vi "AlliGator Phasor Color Map Picker.vi"() -> ()   [LabVIEW 2021, in "AlliGator Phasor Plot Color Map.lvlib"]
doc: "UI to define the vertices of a color map (using cursors) as well as their colors."
uses:
  AlliGator Phasor Plot Color Map.lvlib
  AlliGator Phasor Color Map User Event List.ctl
  5d2066e6-2ae8-4eda-ab8b-78fd27cf9e73.vi
  Phasor/Phasor.lvlib
  Graphs/XY Graph/XY Graph Add-Ons.lvlib
  Error/Error.lvlib
  Arrays/Arrays.lvlib
panel:
  in  "Background":u32(colorbox)=16448250
  in  "Plot Color":u32(colorbox)
  in  "Show Cursor Axes":bool=TRUE
  in  "Decay Range Exponent":dbl=1.0
  in  "Color Array":u32[](array[colorbox])
  out "Color Map Picker Graph":cluster{"X Array":dbl[], "Y Array":dbl[]}[](graph)=[{"X Array"=[1.0, 0.9997482711915926, 0.9989933382359422, 0.9977359612865423, 0.9959774064153977, 0.9937194443381971, 0.9909643486313533, 0.9877148934427036, 0.9839743506981782, 0.9797464868072487, 0.9750355588704727, 0.9698463103929542, 0.9641839665080363, 0.9580542287160347, 0.9514632691433107, 0.9444177243274617, 0.9369246885348925, 0.9289917066174885, 0.9206267664155906, 0.9118382907149164, 0.9026351287655293, 0.8930265473713938, 0.883022221559489, 0.8726322248378774, 0.861867019052535, 0.8507374438531606, 0.8392547057785661, 0.8274303669726426, 0.8152763335422613, 0.8028048435688333, 0.7900284547855991, 0.7769600319330552, 0.7636127338052512, 0.75, 0.7361355373863413, 0.722033306302887, 0.707707506500943, 0.6931725628465641, 0.6784431107959357, 0.6635339816587105, 0.648460187664137, 0.633236906845017, 0.6178794677547131, 0.6024033340325947, 0.5868240888334646, 0.5711574191366419, 0.5554190999505048, 0.5396249784283934, 0.5237909579118704, 0.5079329819174031, 0.4920670180825951, 0.47620904208812787, 0.4603750215716047, 0.4445809000494934, 0.4288425808633563, 0.4131759111665336, 0.39759666596740345, 0.38212053224528514, 0.3667630931549812, 0.35153981233586123, 0.3364660183412878, 0.32155688920406267, 0.30682743715343425, 0.2922924934990553, 0.2779666936971116, 0.2638644626136573, 0.24999999999999878, 0.2363872661947476, 0.22303996806694376, 0.20997154521439987, 0.1971951564311657, 0.18472366645773786, 0.17256963302735667, 0.16074529422143313, 0.1492625561468387, 0.1381329809474643, 0.12736777516212205, 0.1169777784405105, 0.1069734526286058, 0.0973648712344703, 0.08816170928508327, 0.07937323358440912, 0.07100829338251125, 0.06307531146510731, 0.055582275672538095, 0.04853673085668925, 0.041945771283965094, 0.035816033491963606, 0.030153689607045786, 0.02496444112952728, 0.020253513192751316, 0.016025649301821876, 0.012285106557296477, 0.009035651368646702, 0.006280555661802856, 0.004022593584602385, 0.0022640387134577056, 0.0010066617640578368, 0.0002517288084074587, 0.0], "Y Array"=[0.0, 0.015863966749033825, 0.03171195982828225, 0.047528021652091336, 0.06329622678687463, 0.07900069798667494, 0.0946256221802051, 0.1101552663932703, 0.1255739935905396, 0.14086627842071484, 0.15601672284924356, 0.17101007166283436, 0.18583122783016376, 0.20046526770330683, 0.2148974560445858, 0.22911326086370518, 0.24309836805023433, 0.25683869578670315, 0.2703204087277988, 0.28352993193138537, 0.2964539645273202, 0.3090794931103026, 0.3213938048432696, 0.3333845002581458, 0.34503950574105596, 0.3563470856894314, 0.3672958543287666, 0.37787478717712913, 0.3880732321458784, 0.39788092026541605, 0.4072879760251678, 0.41628492731738564, 0.4248627149747572, 0.43301270189221935, 0.4407266817237911, 0.447996887145668, 0.4548159976772593, 0.4611771470522908, 0.4670739301325535, 0.47250040935733434, 0.47745112072203705, 0.4819210792799712, 0.485905784161771, 0.4894012231073895, 0.4924038765061041, 0.49491072094046645, 0.4969192322306272, 0.49842738797597125, 0.49943366959150404, 0.49993706383693753, 0.4999370638369375, 0.4994336695915039, 0.4984273879759711, 0.49691923223062695, 0.4949107209404662, 0.49240387650610384, 0.4894012231073891, 0.48590578416177055, 0.4819210792799707, 0.47745112072203655, 0.4725004093573338, 0.46707393013255283, 0.46117714705229007, 0.4548159976772585, 0.44799688714566727, 0.4407266817237903, 0.43301270189221863, 0.4248627149747565, 0.4162849273173849, 0.40728797602516714, 0.3978809202654153, 0.3880732321458777, 0.3778747871771284, 0.36729585432876594, 0.35634708568943074, 0.34503950574105535, 0.3333845002581452, 0.32139380484326907, 0.30907949311030203, 0.2964539645273197, 0.28352993193138487, 0.27032040872779833, 0.25683869578670276, 0.24309836805023396, 0.22911326086370487, 0.21489745604458552, 0.2004652677033066, 0.18583122783016356, 0.17101007166283425, 0.15601672284924348, 0.14086627842071484, 0.12557399359053964, 0.1101552663932704, 0.09462562218020525, 0.07900069798667515, 0.0632962267868749, 0.04752802165209166, 0.03171195982828264, 0.015863966749034272, 5.053215498074303e-16]}]
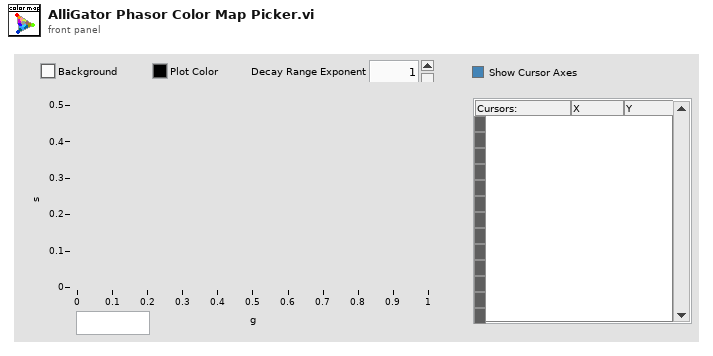
[diagram p1: front panel]
types:
  T1 = typedef "AlliGator Phasor Plot Color Map.lvlib/AlliGator Phasor Color Map User Event List.ctl" = enum16{"Init", "Vertex Update", "Color Change"}
  T2 = typedef "LVCursorListTypeDef.ctl" = cluster{"Name":string, "Color":u32, "Style":u8, "Point Style":u8, "Name Visible":bool, "Allow Drag":bool, "Cursor Mode":u32, "Plot":i32, "Index":i32, "Position":cluster{"X":dbl, "Y":dbl}, "X Scale":u32, "Y Scale":u32, "Watch Plots":i32[], "Watch All Plots":bool, "Plot Area":i32, "Label Offset":cluster{"X":dbl, "Y":dbl}}[]
  T3 = cluster{"Cursor Point Style":u8, "Cursor Style":u8, "Line Style":u8, "Line Width":u8, "Cursor Color":u32}
  T4 = cluster{"Color Array":refnum<vi>, "Color Map Picker Graph":refnum<vi>, "Decay Range Exponent":refnum<vi>}
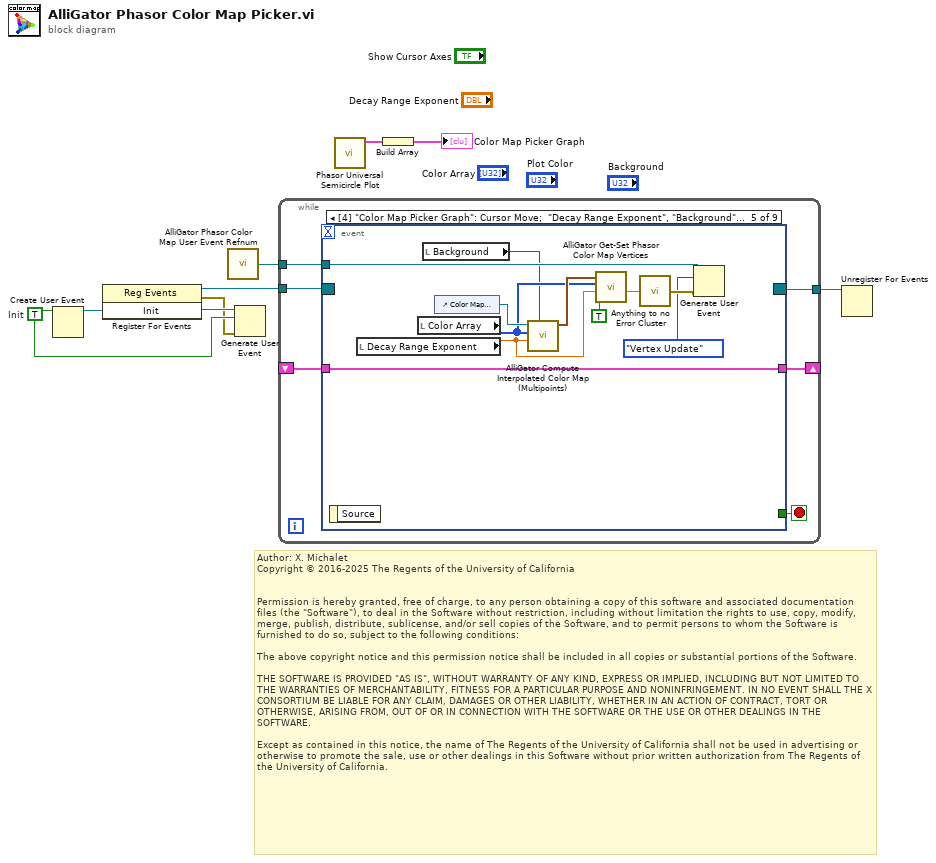
[diagram p0: block diagram]
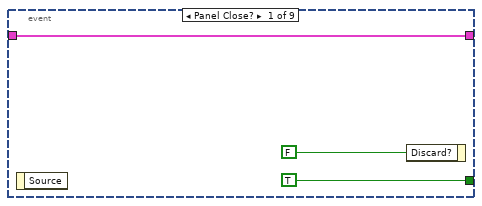
[diagram p2: hidden frame]
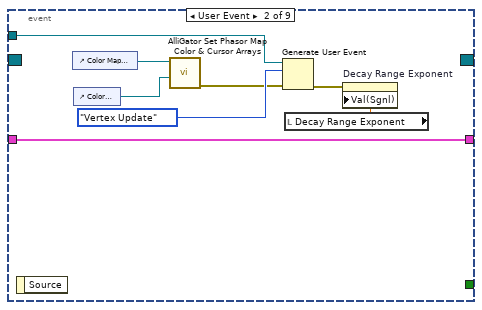
[diagram p3: hidden frame]
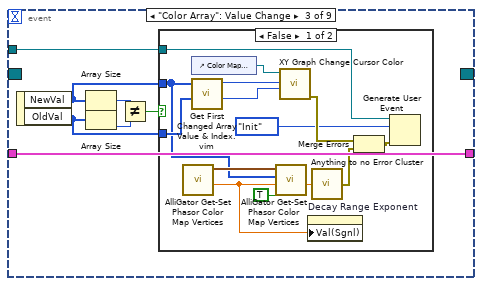
[diagram p4: hidden frame]
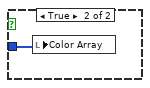
[diagram p5: hidden frame]
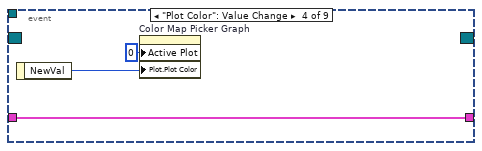
[diagram p6: hidden frame]
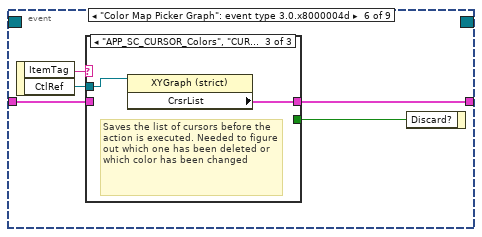
[diagram p7: hidden frame]
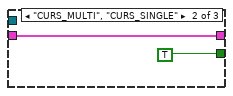
[diagram p9: hidden frame]
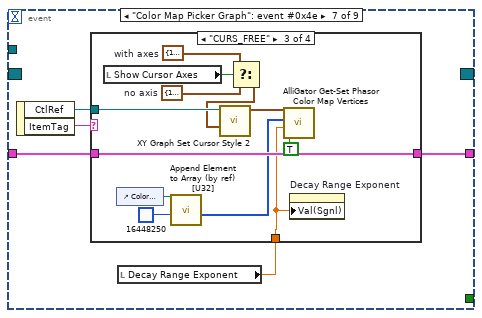
[diagram p10: hidden frame]
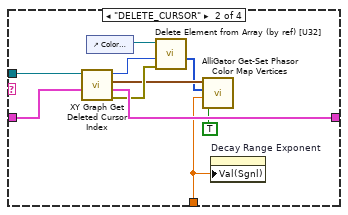
[diagram p12: hidden frame]
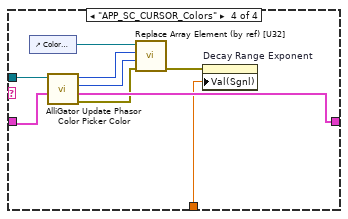
[diagram p13: hidden frame]
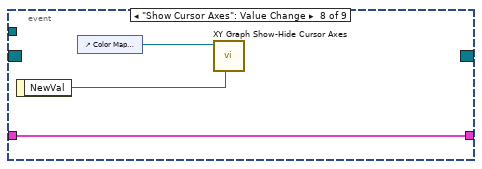
[diagram p14: hidden frame]
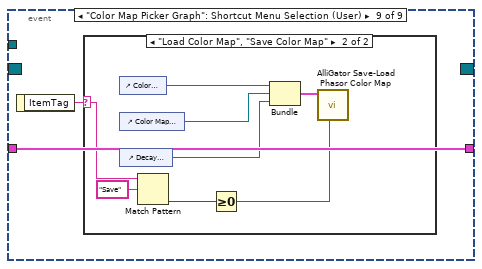
[diagram p15: hidden frame]
diagram:
  w5 = TRUE  # Init
  # "Author: X. Michalet\nCopyright © 2016-2025 The Regents of the University of California\n \n\nPermission is hereby granted, free of charge, to any person obtaining a copy of this software and associated documentation files (the \"Software\"), to deal in the Software without restriction, including without limitation the rights to use, copy, modify, merge, publish, distribute, sublicense, and/or sell copies of the Software, and to permit persons to whom the Software is furnished to do so, subject to the following conditions:\n\nThe above copyright notice and this permission notice shall be included in all copies or substantial portions of the Software.\n\nTHE SOFTWARE IS PROVIDED \"AS IS\", WITHOUT WARRANTY OF ANY KIND, EXPRESS OR IMPLIED, INCLUDING BUT NOT LIMITED TO THE WARRANTIES OF MERCHANTABILITY, FITNESS FOR A PARTICULAR PURPOSE AND NONINFRINGEMENT. IN NO EVENT SHALL THE X CONSORTIUM BE LIABLE FOR ANY CLAIM, DAMAGES OR OTHER LIABILITY, WHETHER IN AN ACTION OF CONTRACT, TORT OR OTHERWISE, ARISING FROM, OUT OF OR IN CONNECTION WITH THE SOFTWARE OR THE USE OR OTHER DEALINGS IN THE SOFTWARE.\n\nExcept as contained in this notice, the name of The Regents of the University of California shall not be used in advertising or otherwise to promote the sale, use or other dealings in this Software without prior written authorization from The Regents of the University of California."
  n1 = Create User Event(user event datatype=w5) -> (user event=w2:refnum<user-event>)  [unwired: 1 in, 1 out]
  n2 = register-events(w2) -> (reference out=w6:refnum<event-registration>, error out=w1:errorcluster)  [unwired: 2 in]
  n3 = call "AlliGator Phasor Color Map User Event Refnum.vi"() -> ("Phasor Color Map Picker Event Refnum"=w3:refnum<user-event>)  [unwired: 9 in]
  n4 = Generate User Event(user event=w2, event data cluster=w5, error in=w1) -> ()  [unwired: 1 in, 2 out]
  n5 = while {
    shift-right: [w13] -> _
    shift-left: _ -> [w12]
    tunnel: w6 -> [w11]
    tunnel: [w10] -> w4
    tunnel: w3 -> [w9]
    stop <- w14 stop-if-true
    n6 = event shown="[4] \"Color Map Picker Graph\": Cursor Move;  \"Decay Range Exponent\", \"Background\": Value Change;  Panel Resize" {
      selector: w11 -> [_ _ _ _ _ _ _ _ _]
      dyn-events: [_ _ _ _ _ _ _ _ _] -> w10
      timeout: _ -> [_ _ _ _ _ _ _ _ _]
      tunnel: [TRUE ("Discard?") _ _ _ _ _ _ _ _] -> w14
      tunnel: [w15 w25 w30 w50 w60 w63 w73 w111 w112] -> w13
      tunnel: w12 -> [w15 w25 w30 w50 w60 w62 w74 w111 w112]
      tunnel: w9 -> [_ w22 w26 _ w53 _ _ _ _]
      event Panel Close? {
        n7 = event-data() -> ()  [unwired: 1 in, 1 out]
        n8 = event-data("Discard?"=FALSE) -> ()  [unwired: 1 in, 1 out]
      }
      event User Event {
        n9 = event-data() -> ()  [unwired: 1 in, 1 out]
        n10 = control-ref of="Color Map Picker Graph"() -> (w24:refnum<vi>)
        n11 = control-ref of="Color Array"() -> (w23:refnum<vi>)
        n12 = call "AlliGator Set Phasor Map Color & Cursor Arrays.vi"("Array in"=w23, "Phasor Graph"=w24) -> ("Error Out"=w20:errorcluster)  [unwired: 9 in]
        n13 = Generate User Event(user event=w22, event data cluster=AlliGator_Phasor_Color_Map_User_Event_List."Vertex Update" ("event data"), error in=w20) -> (error out=w19:errorcluster)  [unwired: 1 in, 1 out]
        n14 = local read "Decay Range Exponent"() -> (w18:dbl)
        n15 = property on="Decay Range Exponent" class="DigNum (strict)"(error in=w19, "Val(Sgnl)"=w18) -> ()  [unwired: 1 in, 2 out]
      }
      event "Color Array": Value Change {
        n16 = event-data() -> ("NewVal"=w27:u32[], "OldVal"=w28:u32[])  [unwired: 1 in]
        n17 = Array Size(array=w27) -> (size(s)=w32:i32)
        n18 = Array Size(array=w28) -> (size(s)=w31:i32)
        n19 = Not Equal?(x=w32, y=w31) -> (x != y?=w29:bool)
        n20 = case shown="False" w29 {
          tunnel: w27 -> [w41 _]
          tunnel: w28 -> [w46 w47]
          tunnel: w26 -> [w35 _]
          frame False {
            n21 = call "AlliGator Get-Set Phasor Color Map Vertices.vi"() -> ("Decay Range Exponent out"=w33:dbl, "Vertices out"=w42:cluster{"X":dbl, "Y":dbl}[])  [unwired: 8 in, 2 out]
            n22 = control-ref of="Color Map Picker Graph"() -> (w45:refnum<vi>)
            n23 = call "Get First Changed Array Value & Index.vim"("OldVal"=w46, "NewVal"=w41) -> ("Changed Value Index"=w43:i32, "Changed Value"=w44:u32)  [unwired: 8 in]
            n24 = call "AlliGator Get-Set Phasor Color Map Vertices.vi"("Set/Get(F)"=TRUE, "Decay Range Exponent in"=w33, "Color Array in"=w41, "Vertices in"=w42) -> ("Decay Range Exponent out"=w37:dbl)  [unwired: 4 in, 3 out]
            n25 = call "XY Graph Change Cursor Color.vi"("Changed Color Index"=w43, "Changed Color"=w44, "XYGraph in"=w45) -> ("Error Out"=w39:errorcluster)  [unwired: 8 in]
            n26 = property on="Decay Range Exponent" class="DigNum (strict)"("Val(Sgnl)"=w33) -> ()  [unwired: 2 in, 2 out]
            n27 = call "Anything to no Error Cluster.vi"("Variant"=w37) -> ("Error Out"=w36:errorcluster)  [unwired: 8 in]
            n28 = Merge Errors(w39, w36) -> (w38:errorcluster)
            n29 = Generate User Event(user event=w35, event data cluster=AlliGator_Phasor_Color_Map_User_Event_List."Init" ("event data"), error in=w38) -> ()  [unwired: 1 in, 2 out]
          }
          frame True {
            n30 = local write "Color Array"(w47) -> ()
          }
        }
      }
      event "Plot Color": Value Change {
        n31 = event-data() -> ("NewVal"=w48:u32)  [unwired: 1 in]
        n32 = property on="Color Map Picker Graph" class="XYGraph (strict)"("Active Plot"=u32 0, "Plot.Plot Color"=w48) -> ()  [unwired: 2 in, 2 out]
      }
      event "Color Map Picker Graph": Cursor Move; "Decay Range Exponent", "Background": Value Change; Panel Resize {
        n33 = event-data() -> ()  [unwired: 1 in, 1 out]
        n34 = local read "Decay Range Exponent"() -> (w56:dbl)
        n35 = local read "Color Array"() -> (w58:u32[])
        n36 = local read "Background"() -> (w51:u32)
        n37 = control-ref of="Color Map Picker Graph"() -> (w61:refnum<vi>)
        n38 = call "AlliGator Compute Interpolated Color Map (Multipoints).vi"("Background Color"=w51, "Decay Range Exponent"=w56, "Color Array"=w58, "XY Graph"=w61) -> ("Vertices"=w59:cluster{"X":dbl, "Y":dbl}[])  [unwired: 6 in, 1 out]
        n39 = call "AlliGator Get-Set Phasor Color Map Vertices.vi"("Set/Get(F)"=TRUE, "Decay Range Exponent in"=w56, "Color Array in"=w58, "Vertices in"=w59) -> ("Decay Range Exponent out"=w55:dbl)  [unwired: 4 in, 3 out]
        n40 = call "Anything to no Error Cluster.vi"("Variant"=w55) -> ("Error Out"=w54:errorcluster)  [unwired: 8 in]
        n41 = Generate User Event(user event=w53, event data cluster=AlliGator_Phasor_Color_Map_User_Event_List."Vertex Update" ("event data"), error in=w54) -> ()  [unwired: 1 in, 2 out]
      }
      event "Color Map Picker Graph": event type 3.0.x8000004d {
        n42 = event-data() -> ("ItemTag"=w66:string, "CtlRef"=w64:refnum<vi>)  [unwired: 1 in]
        n43 = case shown="\"APP_SC_CURSOR_Colors\", \"CURS_FREE\", \"DELETE_CURSOR\"" w66 {
          tunnel: [_ TRUE ("Discard?") _] -> w65
          tunnel: w64 -> [_ _ w71]
          tunnel: [w67 w68 w70] -> w63
          tunnel: w62 -> [w67 w68 _]
          frame "", Default {
          }
          frame "CURS_MULTI", "CURS_SINGLE" {
          }
          frame "APP_SC_CURSOR_Colors", "CURS_FREE", "DELETE_CURSOR" {
            # "Saves the list of cursors before the action is executed. Needed to figure out which one has been deleted or which color has been changed"
            n44 = property class="XYGraph (strict)"(reference=w71) -> ("CrsrList"=w70:T2)  [unwired: 1 in, 2 out]
          }
        }
        n45 = event-data("Discard?"=w65) -> ()  [unwired: 1 in, 1 out]
      }
      event "Color Map Picker Graph": event #0x4e {
        n46 = event-data() -> ("CtlRef"=w75:refnum<vi>, "ItemTag"=w76:string)  [unwired: 1 in]
        n47 = local read "Decay Range Exponent"() -> (w72:dbl)
        n48 = case shown="\"CURS_FREE\"" w76 {
          tunnel: w75 -> [_ w87 w96 w108]
          tunnel: w74 -> [w77 w86 w97 w107]
          tunnel: [w77 w85 w97 w106] -> w73
          tunnel: w72 -> [_ w78 w92 w100]
          frame "", Default {
          }
          frame "DELETE_CURSOR" {
            n49 = call "XY Graph Get Deleted Cursor Index.vi"("Old Cursor List"=w86, "XYGraph in"=w87) -> ("Error Out"=w82:errorcluster, "New Cursor List"=w85:T2, "Vertices"=w81:cluster{"X":dbl, "Y":dbl}[], "Deleted Cursor Index"=w83:i32)  [unwired: 6 in]
            n50 = control-ref of="Color Array"() -> (w84:refnum<vi>)
            n51 = call "Delete Element from Array (by ref) [U32].vi"("Error In"=w82, "Element Index"=w83, "Array in"=w84) -> ("Array w/o Element at Index"=w79:u32[])  [unwired: 6 in, 2 out]
            n52 = call "AlliGator Get-Set Phasor Color Map Vertices.vi"("Set/Get(F)"=TRUE, "Decay Range Exponent in"=w78, "Color Array in"=w79, "Vertices in"=w81) -> ()  [unwired: 4 in, 4 out]
            n53 = property on="Decay Range Exponent" class="DigNum (strict)"("Val(Sgnl)"=w78) -> ()  [unwired: 2 in, 2 out]
          }
          frame "CURS_FREE" {
            w89 = T3 {"Cursor Point Style"=1, "Cursor Style"=0, "Line Style"=2, "Line Width"=0, "Cursor Color"=16448250}  # no axis
            w90 = T3 {"Cursor Point Style"=1, "Cursor Style"=8, "Line Style"=2, "Line Width"=0, "Cursor Color"=16448250}  # with axes
            n54 = local read "Show Cursor Axes"() -> (w91:bool)
            n55 = control-ref of="Color Array"() -> (w99:refnum<vi>)
            n56 = call "Append Element to Array (by ref) [U32].vi"("New Element"=u32 16448250, "Array in"=w99) -> ("Array w New Element"=w94:u32[])  [unwired: 7 in, 2 out]
            n57 = Select(t=w90, s=w91, f=w89) -> (s? t:f=w88:T3)
            n58 = call "XY Graph Set Cursor Style 2.vi"("Cursor Style"=w88, "XYGraph in"=w96) -> ("Vertices"=w95:cluster{"X":dbl, "Y":dbl}[])  [unwired: 8 in, 1 out]
            n59 = call "AlliGator Get-Set Phasor Color Map Vertices.vi"("Set/Get(F)"=TRUE, "Decay Range Exponent in"=w92, "Color Array in"=w94, "Vertices in"=w95) -> ()  [unwired: 4 in, 4 out]
            n60 = property on="Decay Range Exponent" class="DigNum (strict)"("Val(Sgnl)"=w92) -> ()  [unwired: 2 in, 2 out]
          }
          frame "APP_SC_CURSOR_Colors" {
            n61 = control-ref of="Color Array"() -> (w105:refnum<vi>)
            n62 = call "AlliGator Update Phasor Color Picker Color.vi"("New Cursor List in"=w107, "XYGraph in"=w108) -> ("Error Out"=w102:errorcluster, "New Cursor List out"=w106:T2, "Cursor Index"=w103:i32, "Cursor Color"=w104:u32)  [unwired: 6 in]
            n63 = call "Replace Array Element (by ref) [U32].vi"("Error In"=w102, "Index"=w103, "New Element"=w104, "Array in"=w105) -> ("Error Out"=w101:errorcluster)  [unwired: 6 in, 1 out]
            n64 = property on="Decay Range Exponent" class="DigNum (strict)"(error in=w101, "Val(Sgnl)"=w100) -> ()  [unwired: 1 in, 2 out]
          }
        }
      }
      event "Show Cursor Axes": Value Change {
        n65 = event-data() -> ("NewVal"=w109:bool)  [unwired: 1 in]
        n66 = control-ref of="Color Map Picker Graph"() -> (w110:refnum<vi>)
        n67 = call "XY Graph Show-Hide Cursor Axes.vi"("Show Cursor Axes"=w109, "XYGraph in"=w110) -> ()  [unwired: 9 in, 1 out]
      }
      event "Color Map Picker Graph": Shortcut Menu Selection (User) {
        n68 = event-data() -> ("ItemTag"=w113:string)  [unwired: 1 in]
        n69 = case shown="\"Load Color Map\", \"Save Color Map\"" w113 {
          selector: w113 -> [_ w118]
          frame "", Default {
          }
          frame "Load Color Map", "Save Color Map" {
            n70 = control-ref of="Color Array"() -> (w121:refnum<vi>)
            n71 = control-ref of="Color Map Picker Graph"() -> (w120:refnum<vi>)
            n72 = control-ref of="Decay Range Exponent"() -> (w119:refnum<vi>)
            n73 = Match Pattern(string=w118, regular expression="Save") -> (offset past match=w116:i32)  [unwired: 1 in, 3 out]
            n74 = Greater Or Equal To 0?(x=w116) -> (x >= 0?=w115:bool)
            n75 = Bundle("Color Array"=w121, "Color Map Picker Graph"=w120, "Decay Range Exponent"=w119) -> (w114:T4)  [unwired: 1 in]
            n76 = call "AlliGator Save-Load Phasor Color Map.vi"("Save/Load (F)"=w115, "Control References"=w114) -> ()  [unwired: 9 in, 1 out]
          }
        }
      }
    }
  }
  n77 = call "Phasor Universal Semicircle Plot.vi"() -> ("Universal Semi-circle"=w8:cluster{"X Array":dbl[], "Y Array":dbl[]})  [unwired: 9 in, 2 out]
  n78 = Build Array(w8) -> (→"Color Map Picker Graph":cluster{"X Array":dbl[], "Y Array":dbl[]}[])
  n79 = Unregister For Events(event registration refnum=w4) -> ()  [unwired: 1 in, 1 out]
